vi "2 update_currents_drift.vi"   [LabVIEW 2011]
doc: "Finds the error of the boats heading versus movement, and attributes that to current/leeway. This uses the error between heading and bearing, as well as the Think Frequency, to determine the velocity of the currents. Only the current velocity normal to the boat's heading is found, but this is all that we need to know to shift the goal.\n\nTrigonometry is used to isolate the sideways movement of the boat from the total movement of the boat. We then convert this to a velocity, by multiplying by the Think Frequency. This is stored in a trailing average, and set as the Global Absolute Water Current Vector."
uses:
  2 Globals/2 Global.vi
  2 Classes/Angle/Angle.lvclass
  2 Classes/Angle/directionOfRotation.ctl
  2 Classes/Vectors/CartesianVectors/CartesianVector/CartesianVector.lvclass
types:
  T1 = typedef "Angle.lvclass/directionOfRotation.ctl" = enum16{"Clockwise", "Counter-Clockwise"}
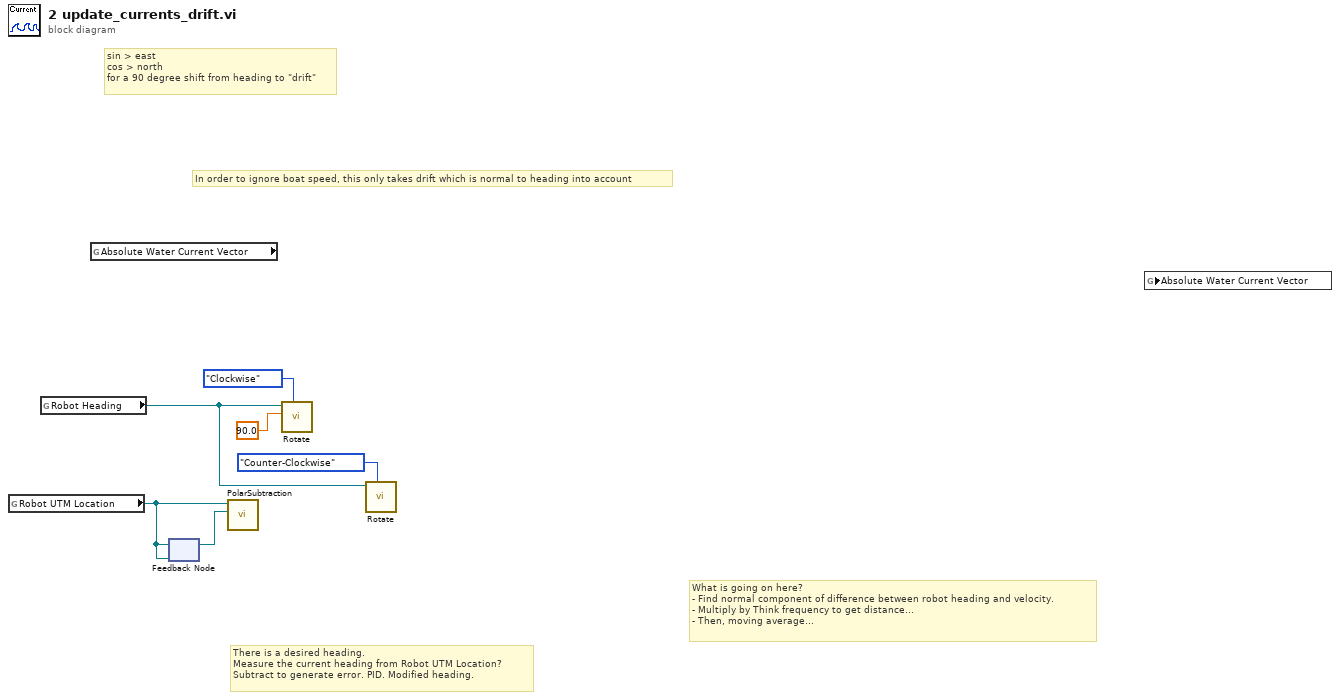
[diagram p0: block diagram]
diagram:
  # "What is going on here?\n- Find normal component of difference between robot heading and velocity.\n- Multiply by Think frequency to get distance...\n- Then, moving average..."
  # "There is a desired heading.\nMeasure the current heading from Robot UTM Location?\nSubtract to generate error. PID. Modified heading."
  # "sin > east\ncos > north\nfor a 90 degree shift from heading to \"drift\""
  # "In order to ignore boat speed, this only takes drift which is normal to heading into account"
  n1 = global read "2 Global.vi" "Robot UTM Location"() -> (w3:refnum<class "UTM_Location.lvclass">)
  n2 = global read "2 Global.vi" "Robot Heading"() -> (w2:refnum<class "Angle.lvclass">)
  n3 = global read "2 Global.vi" "Absolute Water Current Vector"() -> ()  [unwired: 1 out]
  n4 = feedback #1(w3) -> (w4:refnum<class "UTM_Location.lvclass">)
  n5 = feedback-in #1(w3) -> ()
  n6 = call "PolarSubtraction.vi"("CartesianVector 2"=w4, "CartesianVector 1"=w3) -> ()  [unwired: 8 in, 2 out]
  n7 = call "Rotate.vi"("Direction of Rotation"=directionOfRotation."Clockwise", "Rotation Angle (Deg.)"=90.0, "Angle in"=w2) -> ()  [unwired: 6 in, 3 out]
  n8 = call "Rotate.vi"("Direction of Rotation"=directionOfRotation."Counter-Clockwise", "Angle in"=w2) -> ()  [unwired: 7 in, 3 out]
  n9 = global read "2 Global.vi" "Absolute Water Current Vector"() -> ()  [unwired: 1 in]
